vi "Launch.vi"(0 "Caller Interface":refnum<class "Actor Interface.lvclass">, 1 "Loggers":refnum<class "Logger.lvclass">[](array[class]) caption="Loggers (none)", 5 "Error in":errorcluster caption="Error in (no error)") -> (14 "Actor Interface":refnum<class "Actor Interface.lvclass">, 15 "Actor Name":string="Module", 19 "Error out":errorcluster)   [LabVIEW 2019, in "GP Module.lvlib"]
doc: "<Developer>\nGPower\n22/9 2019"
uses:
  <vilib>/GPower/Logger/Library/Logger Class/Logger.lvclass
  <vilib>/GPower/Actor/Library/Actor Interface Class/Actor Interface.lvclass
  Actors/Module/Module Class/Module.lvclass
  C:/Program Files (x86)/National Instruments/LabVIEW 2019/vi.lib/GPower/Actor/Library/Actor Class/Actor.lvclass
  Actors/Module/GP Module.lvlib
  <vilib>/GPower/Actor/Library/Actor Class/Actor.lvclass
  <vilib>/GPower/UI/Library/GP UI.lvlib
panel:
  in  "Boolean":bool
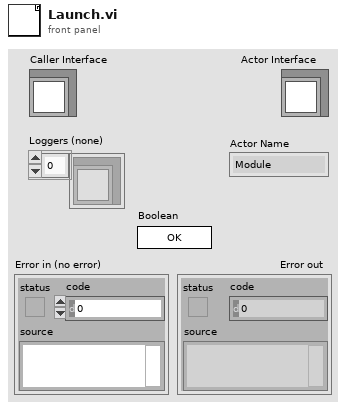
[diagram p1: front panel]
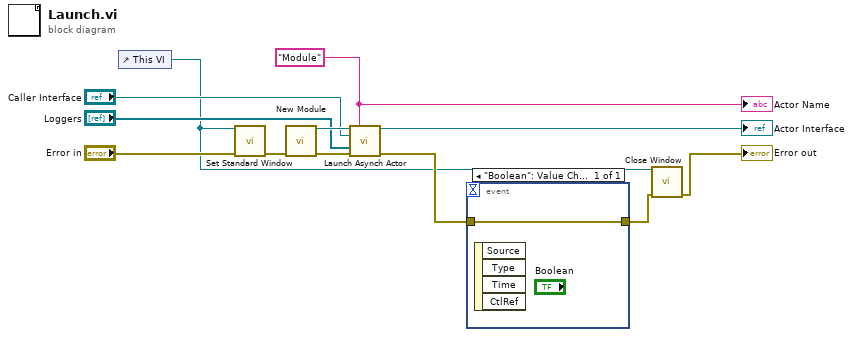
[diagram p0: block diagram]
diagram:
  w11 = "Module" ("Actor Name")
  n1 = control-ref of="This VI"() -> (w1:refnum<vi>)
  n2 = call <vilib>:"Set Standard Window.vi"("VI Refnum"=w1, "Error in"="Error in") -> ("Error out"=w5:errorcluster)  [unwired: 13 in]
  n3 = call "New Module.vi"("Error in"=w5) -> ("New Module"=w12:refnum<class "Module.lvclass">, "Error out"=w10:errorcluster)  [unwired: 13 in]
  n4 = call <vilib>:"Launch Asynch Actor.vi"("Actor"=w12, "Actor Name"=w11, "Caller Interface"="Caller Interface", "Loggers"="Loggers", "Error in"=w10) -> ("Actor Interface"=→"Actor Interface":refnum<class "Actor Interface.lvclass">, "Error out"=w4:errorcluster)  [unwired: 9 in]
  n5 = event shown="[0] \"Boolean\": Value Change" {
    selector: _ -> [_]
    dyn-events: _ -> [_]
    timeout: _ -> [_]
    tunnel: w4 -> [w13]
    tunnel: [w13] -> w3
    event "Boolean": Value Change {
      n6 = event-data() -> ()  [unwired: 1 in, 4 out]
    }
  }
  n7 = call <vilib>:"Close Window.vi"("VI Refnum"=w1, "Error in"=w3) -> ("Error out"=→"Error out":errorcluster)  [unwired: 13 in]
  "Actor Name" <- w11
